vi "Serializer Factory.vi"(5 "Display Format":T1) -> (2 "Serializer":refnum<class "Serializer.lvclass">)   [LabVIEW 2017, in "Error Log.lvlib"]
uses:
  Error Log.lvlib
  Type Defs/Display Format.ctl
  Serializer/Serializer.lvclass
  Serializer.PlainText/Serializer.PlainText.lvclass
  \\192.168.1.40\Neosoft/Partage/Dossiers Personnels/BRO/DevTools_BR/wc/ErrorLog/src/Serializer/Serializer.lvclass
  Serializer.XML/Serializer.XML.lvclass
  Serializer.JSON/Serializer.JSON.lvclass
  Serializer.PlainText.INI/Serializer.PlainText.INI.lvclass
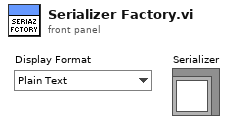
[diagram p1: front panel]
types:
  T1 = typedef "Error Log.lvlib/Display Format.ctl" = enum16{"Plain Text", "INI", "XML", "JSON"}
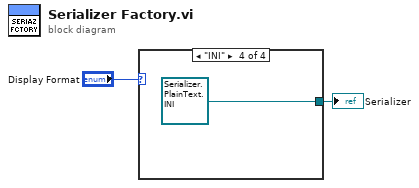
[diagram p0: block diagram]
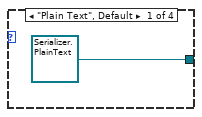
[diagram p2: hidden frame]
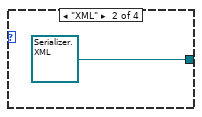
[diagram p3: hidden frame]
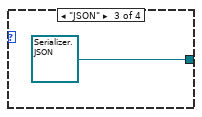
[diagram p4: hidden frame]
diagram:
  n1 = case shown="\"INI\"" "Display Format" {
    tunnel: [refnum<class "Serializer.PlainText.lvclass"> refnum ("Error Log.lvlib:Serializer.PlainText.lvclass") refnum<class "Serializer.XML.lvclass"> refnum ("Error Log.lvlib:Serializer.XML.lvclass") refnum<class "Serializer.JSON.lvclass"> refnum ("Error Log.lvlib:Serializer.JSON.lvclass") refnum<class "Serializer.PlainText.INI.lvclass"> refnum ("Error Log.lvlib:Serializer.PlainText.INI.lvclass")] -> w1
    frame "Plain Text", Default {
    }
    frame "XML" {
    }
    frame "JSON" {
    }
    frame "INI" {
    }
  }
  "Serializer" <- w1
